vi "SettingsWks.vi"(2 "Path":path, 3 "Origin.IOApplication":refnum<k7>) -> (0 "SettingsWks":refnum<k7>, 1 "Origin.IOApplication":refnum<k7>)   [LabVIEW 2014]
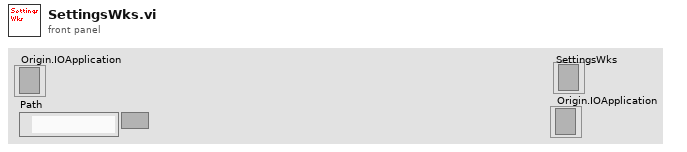
[diagram p1: front panel]
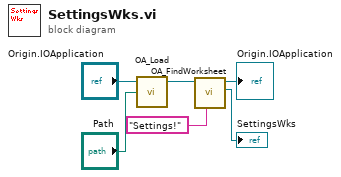
[diagram p0: block diagram]
diagram:
  n1 = call <vilib>:"OA_Load.vi"("Path"="Path", "Origin.IOApplication"="Origin.IOApplication") -> ("Origin.IOApplication"=w6:refnum<k7>)  [unwired: 1 in, 2 out]
  n2 = call <vilib>:"OA_FindWorksheet.vi"("Name"="Settings!", "Origin.IOApplication"=w6) -> ("Origin.Worksheet"=→"SettingsWks":refnum<k7>, "Origin.IOApplication"=→"Origin.IOApplication":refnum<k7>)  [unwired: 7 in, 1 out]
